vi "IAmGLF-NotARefnum.vi"(11 "Engine in":refnum<class "Engine.lvclass">) -> (2 "Not A Valid Refnum?":bool=TRUE, 3 "Engine out":refnum<class "Engine.lvclass">)   [LabVIEW 2024, in "GLF.lvlib" / "Engine.lvclass"]
doc: "<B>Summary</B>\nReturns <B>True</B> if the class is invalid."
uses:
  Engine.lvclass
  Engine.lvclass/Engine.ctl
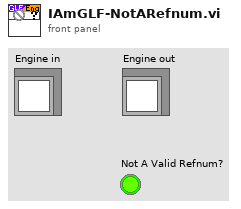
[diagram p1: front panel]
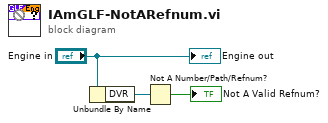
[diagram p0: block diagram]
diagram:
  n1 = Unbundle By Name("Engine in") -> ("DVR"=w1:refnum<data-value>)
  n2 = Not A Number/Path/Refnum?(number/path/refnum=w1) -> (NaN/Path/Refnum?=→"Not A Valid Refnum?":bool)
  "Engine out" <- "Engine in"
